vi "Get Smart GFI.vi"(8 "error IO":errorcluster, 11 "VISA resource name":refnum<visa-resource-name>) -> (0 "error Out":errorcluster, 1 "Smart GFI":dbl, 2 "Smart GFI?":bool, 3 "VISA resource Out":refnum<visa-resource-name>)   [LabVIEW 2012, in "Associated Research 78XX Series.lvlib"]
uses:
  <instrlib>/Associated Research 78XX Series/Associated Research 78XX Series.lvlib
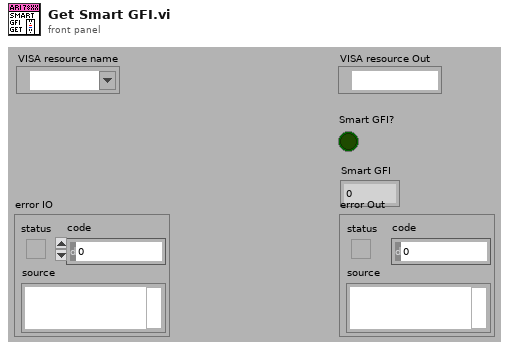
[diagram p1: front panel]
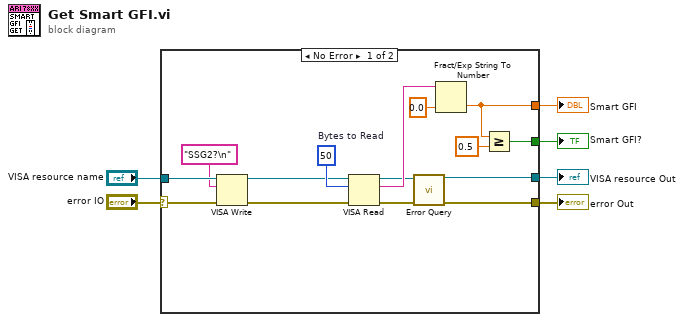
[diagram p0: block diagram]
diagram:
  n1 = case shown="No Error" "error IO" {
    selector: "error IO" -> [w21 w23]
    tunnel: [w18 w23] -> w2
    tunnel: [w19 w22] -> w4
    tunnel: "VISA resource name" -> [w20 w22]
    tunnel: [w10 _] -> w3
    tunnel: [w9 _] -> w1
    frame No Error {
      w14 = u32 50  # Bytes to Read
      n2 = VISA Write(VISA resource name=w20, write buffer="SSG2?\n" ("Command to Send (empty)"), error in (no error)=w21) -> (VISA resource name out=w8:refnum<visa-resource-name>, error out=w7:errorcluster)  [unwired: 1 out]
      n3 = VISA Read(VISA resource name=w8, byte count=w14, error in (no error)=w7) -> (VISA resource name out=w13:refnum<visa-resource-name>, read buffer=w16:string, error out=w12:errorcluster)  [unwired: 1 out]
      n4 = call <instrlib>:"Error Query.vi"("VISA resource name"=w13, "error in (no error)"=w12) -> ("VISA resource name out"=w19:refnum<visa-resource-name>, "error out"=w18:errorcluster)  [unwired: 10 in, 2 out]
      n5 = Fract/Exp String To Number(string=w16, default (0 dbl)=0.0 ("default (0 DBL)")) -> (number=w10:dbl)  [unwired: 2 in, 1 out]
      n6 = Greater Or Equal?(x=w10, y=0.5 ("x")) -> (x >= y?=w9:bool)
    }
    frame Error {
    }
  }
  "VISA resource Out" <- w4
  "Smart GFI" <- w3
  "error Out" <- w2
  "Smart GFI?" <- w1
